vi "setup ADC LV.vi"(9 "adcSetting":u8, 10 "adcNum":u8, 11 "instance":i32) -> (3 "function return":u32)   [LabVIEW 2025, in "SADI_FW3.lvlib"]
doc: "SADI_API_Wrapper unsigned int setupADC_LV( int instance ,\n uint8_t adcNum ,\n uint8_t adcSetting );"
uses:
  SADI_FW3.lvlib
  SADI_FW3.dll
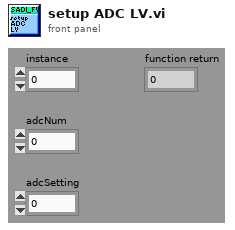
[diagram p1: front panel]
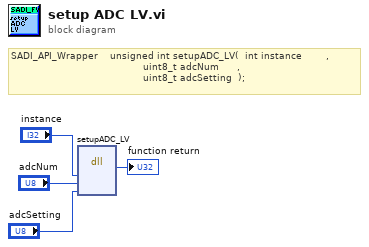
[diagram p0: block diagram]
diagram:
  # "SADI_API_Wrapper    unsigned int setupADC_LV(  int instance        ,\n                                            uint8_t adcNum      ,\n                                            uint8_t adcSetting  );"
  n1 = dll-call lib="C:/Users/noaht/School/Fall 2025/Controls Lab/Lab 3/EML4314c_FA25_framework_0/LVLib/SADI_FW3.*" fn="setupADC_LV"("instance"="instance", "adcNum"="adcNum", "adcSetting"="adcSetting") -> (→"function return":u32)  [unwired: 6 in, 2 out]
